vi "StellarNet Get Operating Parameters from XML.vi"(8 "error in (no error)":errorcluster, 11 "XML File Path":path) -> (0 "error out":errorcluster, 2 "file or folder exists?":bool, 3 "Operating Parameters":T1(array[cluster]) {"Digitizer Clock Rate Setting" min=1 max=3; "Optical Smoothing Level" min=0 max=4 step=1; "Number of Scans to Average" min=1 max=10000 step=1})   [LabVIEW 2023]
uses:
  <vilib>/Utility/xml.llb/Read From XML File(string).vi
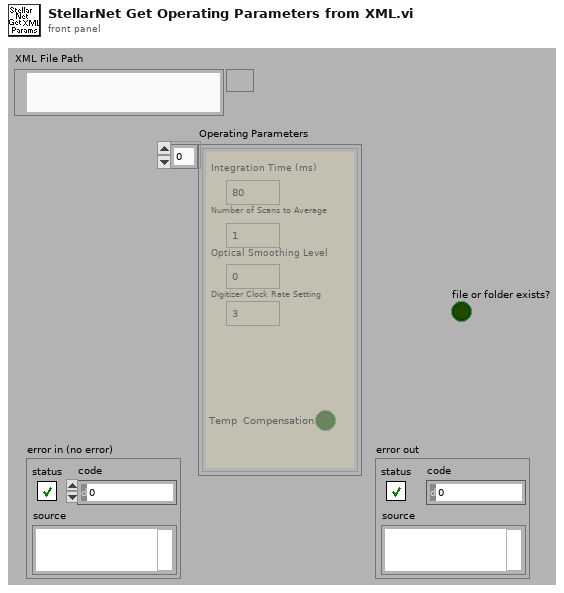
[diagram p1: front panel]
types:
  T1 = cluster{"Integration Time (ms)":i32, "Number of Scans to Average":i32, "Optical Smoothing Level":i32, "Digitizer Clock Rate Setting":i32, "Temp  Compensation ":bool}[]
  T2 = cluster{"Integration Time (ms)":i32, "Number of Scans to Average":i32, "Optical Smoothing Level":i32, "Digitizer Clock Rate Setting":i32, "Drift Correct":bool}[]
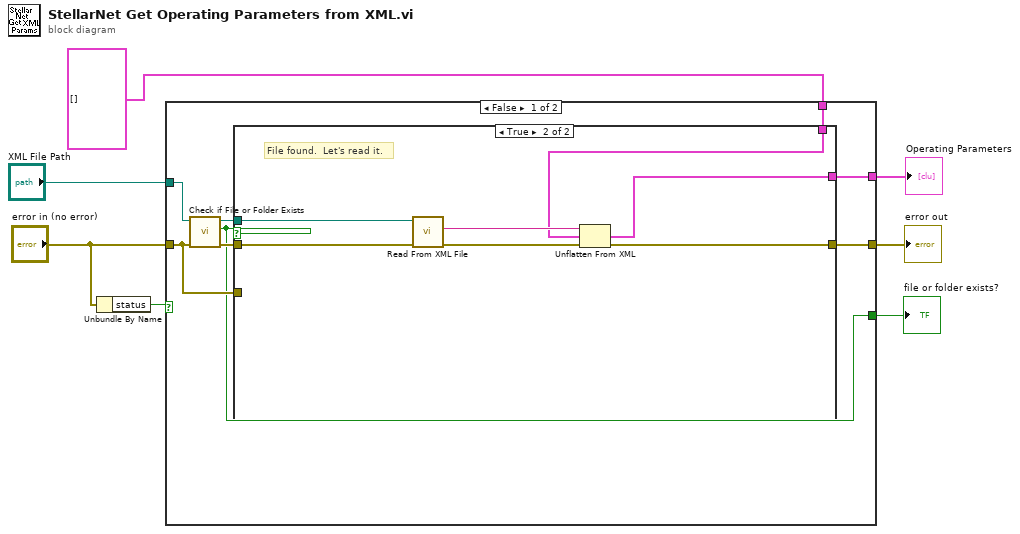
[diagram p0: block diagram]
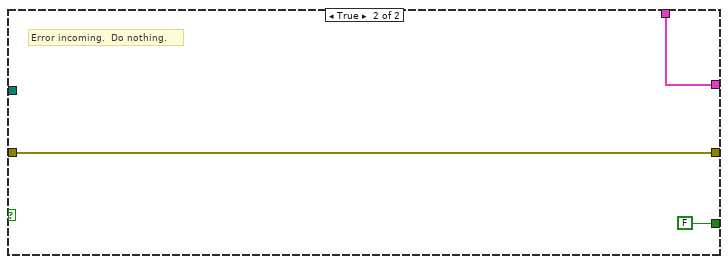
[diagram p3: hidden frame]
diagram:
  n1 = Unbundle By Name("error in (no error)") -> ("status"=w5:bool)
  n2 = case shown="False" w5 {
    tunnel: "XML File Path" -> [w15 _]
    tunnel: "error in (no error)" -> [w11 w27]
    tunnel: [w12 w27] -> w6
    tunnel: [w10 w26] -> w1
    tunnel: T2 [] ("Operating Parameters") -> [w9 w26]
    tunnel: [w8 FALSE ("file or folder exists?")] -> w3
    frame False {
      n3 = call <vilib>:"Check if File or Folder Exists.vi"("error in (no error)"=w11, "path"=w15) -> ("error out"=w14:errorcluster, "file or folder exists?"=w8:bool, "dup path"=w13:path)  [unwired: 7 in]
      n4 = case shown="True" w8 {
        tunnel: w14 -> [_ w22]
        tunnel: [w17 w21] -> w12
        tunnel: w13 -> [_ w20]
        tunnel: w11 -> [w17 _]
        tunnel: [w16 w19] -> w10
        tunnel: w9 -> [w16 w18]
        frame False {
          # "File not found.  We'll create one later, so just pass the incoming error cluster through."
        }
        frame True {
          # "File found.  Let's read it."
          n5 = call-poly <vilib>:"Read From XML File.vi"("error in (no error)"=w22, "XML File Path"=w20) -> ("error out"=w23:errorcluster, "XML Elements"=w24:string)  [unwired: 7 in, 1 out]
          n6 = Unflatten From XML(xml string=w24, type=w18, error in (no error)=w23) -> (value=w19:T2, error out=w21:errorcluster)
        }
      }
    }
    frame True {
      # "Error incoming.  Do nothing."
    }
  }
  "error out" <- w6
  "Operating Parameters" <- w1
  "file or folder exists?" <- w3
